vi "Rename AF Message.vi"() -> ()   [LabVIEW 2020]
uses:
  <vilib>/Utility/traverseref.llb/TRef TravTarget.ctl
  <vilib>/Utility/traverseref.llb/VI Scripting - Traverse.lvlib
  <vilib>/Utility/EditLVLibs/Edit LVLibs.lvlib
panel:
  in  "Cancel Button":bool
  in  "OK Button":bool
  in  "Update Actor VI name as well? (F)":bool
  in  "New Name (leave off the \" Msg.lvclass\" part)":string
  in  "Message to rename":path
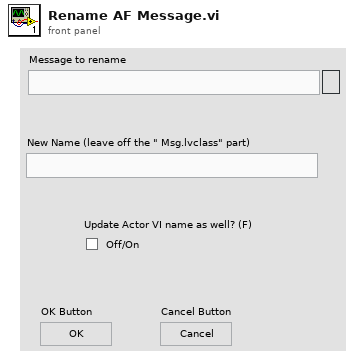
[diagram p1: front panel]
types:
  T1 = typedef "TRef TravTarget.ctl" = enum16{"FP", "BD", "Other"}
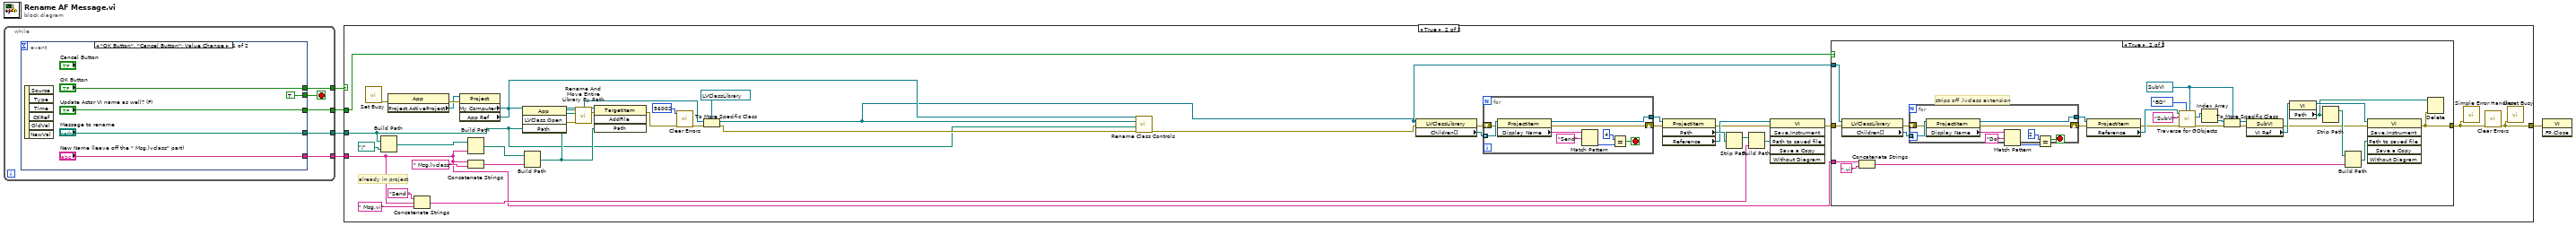
[diagram p0: block diagram]
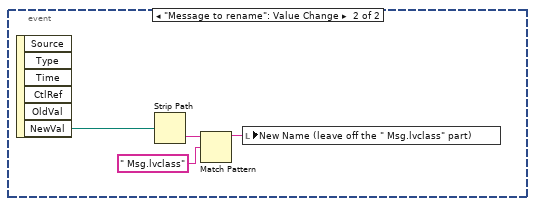
[diagram p2: hidden frame]
diagram:
  n1 = while {
    tunnel: [w10] -> w5
    tunnel: [w9] -> w4
    tunnel: [w8] -> w3
    tunnel: [w7] -> w2
    stop <- w6 stop-if-true
    n2 = event shown="[0] \"OK Button\", \"Cancel Button\": Value Change" {
      selector: _ -> [_ _]
      dyn-events: _ -> [_ _]
      timeout: _ -> [_ _]
      tunnel: ["OK Button" _] -> w10
      tunnel: ["Update Actor VI name as well? (F)" _] -> w9
      tunnel: ["New Name (leave off the \" Msg.lvclass\" part)" _] -> w8
      tunnel: ["Message to rename" _] -> w7
      tunnel: [TRUE _] -> w6
      event "OK Button", "Cancel Button": Value Change {
        n3 = event-data() -> ()  [unwired: 1 in, 6 out]
      }
      event "Message to rename": Value Change {
        n4 = event-data() -> ("NewVal"=w19:path)  [unwired: 1 in, 5 out]
        n5 = Strip Path(path=w19) -> (name=w18:string)  [unwired: 1 out]
        n6 = Match Pattern(string=w18, regular expression=" Msg.lvclass") -> (before substring=w16:string)  [unwired: 1 in, 3 out]
        n7 = local write "New Name (leave off the \" Msg.lvclass\" part)"(w16) -> ()
      }
    }
  }
  n8 = case shown="True" w5 {
    tunnel: w2 -> [_ w21]
    tunnel: w3 -> [_ w38]
    tunnel: w4 -> [_ w37]
    tunnel: [_ w24] -> w1
    frame False {
    }
    frame True {
      # "already in project"
      n9 = call <vilib>:"Set Busy.vi"() -> ("error out"=w27:errorcluster)  [unwired: 10 in, 1 out]
      n10 = Build Path(base path=w21, name or relative path=path "../..") -> (appended path=w56:path)
      n11 = property class="App"(error in=w27) -> (error out=w34:errorcluster, "Project.ActiveProject"=w28:refnum<vi>)  [unwired: 1 in, 1 out]
      n12 = Concatenate Strings("Send " ("string"), w38, " Msg.vi" ("string")) -> (w43:string)
      n13 = property class="Project"(reference=w28, error in=w34) -> ("My Computer"=w33:refnum<vi>, "App Ref"=w23:refnum<vi>)  [unwired: 2 out]
      n14 = Build Path(base path=w56, name or relative path=w38) -> (appended path=w55:path)
      n15 = Concatenate Strings(w38, " Msg.lvclass" ("string")) -> (w54:string)
      n16 = invoke class="App" method="LVClass.Open"(reference=w23, "Path"=w21) -> (error out=w30:errorcluster, "LVClass.Open"=w59:refnum<vi>)  [unwired: 2 in, 2 out]
      n17 = Build Path(base path=w55, name or relative path=w54) -> (appended path=w52:path)
      n18 = call <vilib>:"Rename And Move Entire Library By Path.vi"("error in (no error)"=w30, "New library path"=w52, "Library ref in"=w59) -> ("error out"=w26:errorcluster, "Library ref out"=w31:refnum<vi>)  [unwired: 7 in]
      n19 = invoke class="TargetItem" method="AddFile"(reference=w33, error in=w26, "Path"=w52) -> (error out=w35:errorcluster)  [unwired: 1 in, 3 out]
      n20 = call <vilib>:"Clear Errors.vi"("error in (no error)"=w35, "specific error code to clear (0: all)"=56002) -> ("error out"=w25:errorcluster)  [unwired: 4 in, 1 out]
      n21 = To More Specific Class(target class=refnum<vi> refnum ("Class in"), reference=w31, error in=w25) -> (specific class reference=w20:refnum<vi>, error out=w22:errorcluster)
      n22 = call "Rename Class Controls.vi"("error in (no error)"=w22, "Old Class"=w21, "Class to Rename"=w20, "App Ref"=w23) -> ("error out"=w58:errorcluster)  [unwired: 7 in]
      n23 = property class="LVClassLibrary"(reference=w20, error in=w58) -> (error out=w50:errorcluster, "Children[]"=w51:refnum<vi>[])  [unwired: 1 out]
      n24 = for {
        tunnel: w51 -> [w104] mode=indexing
        shift-right: [w100] -> w42
        shift-left: w50 -> [w101]
        tunnel: [w99] -> w49
        stop <- w97 stop-if-true
        n25 = property class="ProjectItem"(reference=w104, error in=w101) -> (reference out=w99:refnum<vi>, error out=w100:errorcluster, "Display Name"=w98:string)
        n26 = Match Pattern(string=w98, regular expression="Send") -> (offset past match=w102:i32)  [unwired: 1 in, 3 out]
        n27 = Equal?(x=4, y=w102) -> (x = y?=w97:bool)
      }
      n28 = property class="ProjectItem"(reference=w49, error in=w42) -> (error out=w41:errorcluster, "Path"=w48:path, "Reference"=w46:refnum<vi>)  [unwired: 1 out]
      n29 = Strip Path(path=w48) -> (stripped path=w47:path)  [unwired: 1 out]
      n30 = Build Path(base path=w47, name or relative path=w43) -> (appended path=w40:path)
      n31 = invoke class="VI" method="Save.Instrument"(reference=w46, error in=w41, "Path to saved file"=w40) -> (error out=w39:errorcluster)  [unwired: 3 in, 5 out]
      n32 = case shown="True" w37 {
        tunnel: w39 -> [w60 w63]
        tunnel: [w60 w62] -> w29
        tunnel: w38 -> [_ w73]
        tunnel: w20 -> [_ w66]
        frame False {
        }
        frame True {
          w79 = refnum<vi> refnum ("Other Refnum")
          # "strips off .lvclass extension"
          n33 = property class="LVClassLibrary"(reference=w66, error in=w63) -> (error out=w69:errorcluster, "Children[]"=w70:refnum<vi>[])  [unwired: 1 out]
          n34 = Concatenate Strings(w73, ".vi" ("string")) -> (w71:string)
          n35 = for {
            tunnel: w70 -> [w95] mode=indexing
            shift-right: [w91] -> w67
            shift-left: w69 -> [w92]
            tunnel: [w90] -> w68
            stop <- w88 stop-if-true
            n36 = property class="ProjectItem"(reference=w95, error in=w92) -> (reference out=w90:refnum<vi>, error out=w91:errorcluster, "Display Name"=w89:string)
            n37 = Match Pattern(string=w89, regular expression="Do") -> (offset past match=w93:i32)  [unwired: 1 in, 3 out]
            n38 = Equal?(x=2, y=w93) -> (x = y?=w88:bool)
          }
          n39 = property class="ProjectItem"(reference=w68, error in=w67) -> (error out=w64:errorcluster, "Reference"=w65:refnum<vi>)  [unwired: 1 out]
          n40 = call <vilib>:"Traverse for GObjects.vi"("Other Refnum"=w79, "Traverse Target"=TRef_TravTarget."BD", "error in (no error)"=w64, "Class Name"="SubVI", "VI Refnum"=w65) -> ("error out"=w84:errorcluster, "References"=w83:refnum<vi>[])  [unwired: 3 in, 2 out]
          n41 = Index Array(array=w83) -> (element=w81:refnum<vi>)  [unwired: 1 in]
          n42 = To More Specific Class(target class=w79, reference=w81, error in=w84) -> (specific class reference=w80:refnum<vi>, error out=w82:errorcluster)
          n43 = property class="SubVI"(reference=w80, error in=w82) -> (error out=w74:errorcluster, "VI Ref"=w78:refnum<vi>)  [unwired: 1 out]
          n44 = property class="VI"(reference=w78) -> (reference out=w77:refnum<vi>, "Path"=w61:path)  [unwired: 1 in, 1 out]
          n45 = Strip Path(path=w61) -> (stripped path=w76:path)  [unwired: 1 out]
          n46 = Build Path(base path=w76, name or relative path=w71) -> (appended path=w75:path)
          n47 = invoke class="VI" method="Save.Instrument"(reference=w77, error in=w74, "Path to saved file"=w75) -> (error out=w62:errorcluster)  [unwired: 3 in, 5 out]
          n48 = Delete(path (use dialog)=w61, error in=w62) -> ()  [unwired: 3 in, 3 out]
        }
      }
      n49 = call <vilib>:"Simple Error Handler.vi"("error in (no error)"=w29) -> ()  [unwired: 4 in, 5 out]
      n50 = call <vilib>:"Clear Errors.vi"("error in (no error)"=w29) -> ("error out"=w24:errorcluster)  [unwired: 5 in, 1 out]
      n51 = call <vilib>:"Unset Busy.vi"("error in (no error)"=w24) -> ()  [unwired: 10 in, 1 out]
    }
  }
  n52 = invoke class="VI" method="FP.Close"(error in=w1) -> ()  [unwired: 2 in, 3 out]
